vi "Savitzky-Golay Filter (CDB).vi"(8 "Weight":dbl[](array[numeric]), 9 "polynomial order":i32=3, 10 "side points":i32=6, 11 "X":cdb[](array[numeric])) -> (0 "error":i32, 3 "Filtered X":cdb[](array[numeric]))   [LabVIEW 2020, in "NI_AALBase.lvlib"]
doc: "Filters the input data sequence<B> X</B> using a Savitzky-Golay FIR smoothing filter. Wire data to the <B>X</B> input to determine the polymorphic instance to use or manually select the instance."
uses:
  NI_AALBase.lvlib
panel:
  # "Savitzky-Golay Filter"
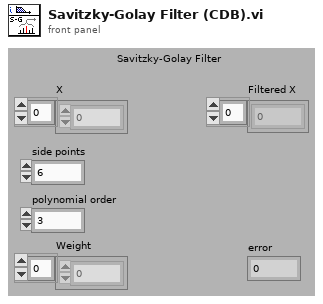
[diagram p1: front panel]
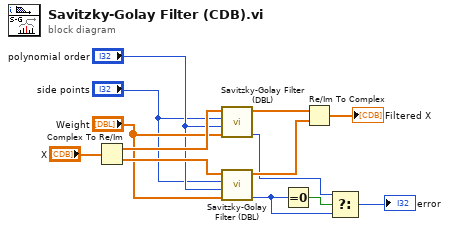
[diagram p0: block diagram]
diagram:
  n1 = Complex To Re/Im(x + iy="X") -> (x=w12:dbl[], y=w11:dbl[])
  n2 = call "Savitzky-Golay Filter (DBL).vi"("Weight"="Weight", "polynomial order"="polynomial order", "side points"="side points", "X"=w12) -> ("error"=w5:i32, "Filtered X"=w9:dbl[])  [unwired: 6 in]
  n3 = call "Savitzky-Golay Filter (DBL).vi"("Weight"="Weight", "polynomial order"="polynomial order", "side points"="side points", "X"=w11) -> ("error"=w4:i32, "Filtered X"=w8:dbl[])  [unwired: 6 in]
  n4 = Equal To 0?(x=w4) -> (x = 0?=w6:bool)
  n5 = Re/Im To Complex(1:w8, 2:w9) -> (0:→"Filtered X":cdb[])
  n6 = Select(t=w5, s=w6, f=w4) -> (s? t:f=→"error":i32)
